vi "Vertical Aiming Calculator.vi"() -> ()   [LabVIEW 2015]
uses:
  <vilib>/Utility/file.llb/Write Delimited Spreadsheet (DBL).vi
panel:
  in  "Robot Constants":T1={"Distance from Pivot Point to Drive Mount(in)"=2.0, "Distance from Pivot Point to Arm Mount(in)"=2.0}
  in  "Other Constants":T2={"Ball Diameter(in)"=10.0, "Air Density(g/in^3)"=0.02, "Drag coefficient"=0.5, "Ball Mass(g)"=300.0, "gravity(in/s^2)"=-386.09, "Minimum Goal Height(in)"=90.0, "Maximum Goal Height(in)"=104.0}
  in  "Sims/angle":i32
  in  "Min Angle":i32
  in  "Max Angle":i32
  in  "Initial Velocity":dbl
  in  "Framerate":i32
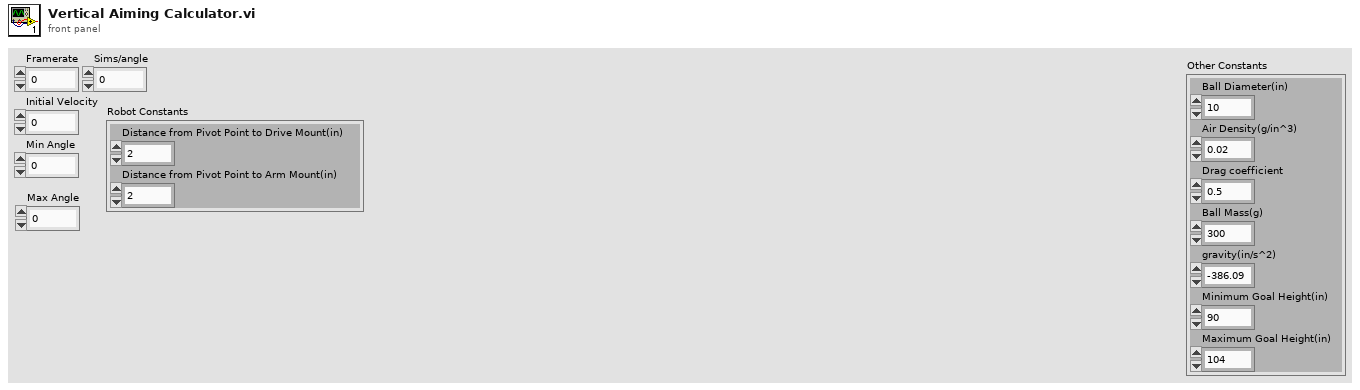
[diagram p1: front panel]
types:
  T1 = cluster{"Distance from Pivot Point to Drive Mount(in)":dbl, "Distance from Pivot Point to Arm Mount(in)":dbl}
  T2 = cluster{"Ball Diameter(in)":dbl, "Air Density(g/in^3)":dbl, "Drag coefficient":dbl, "Ball Mass(g)":dbl, "gravity(in/s^2)":dbl, "Minimum Goal Height(in)":dbl, "Maximum Goal Height(in)":dbl}
  T3 = cluster{"Firing Angle":dbl, "Framerate":dbl, "Initial Velocity":dbl}
  T4 = cluster{"Minimum Distance":dbl, "Ideal Distance":dbl, "Viable Distances":dbl[], "Maximum Distance":dbl}
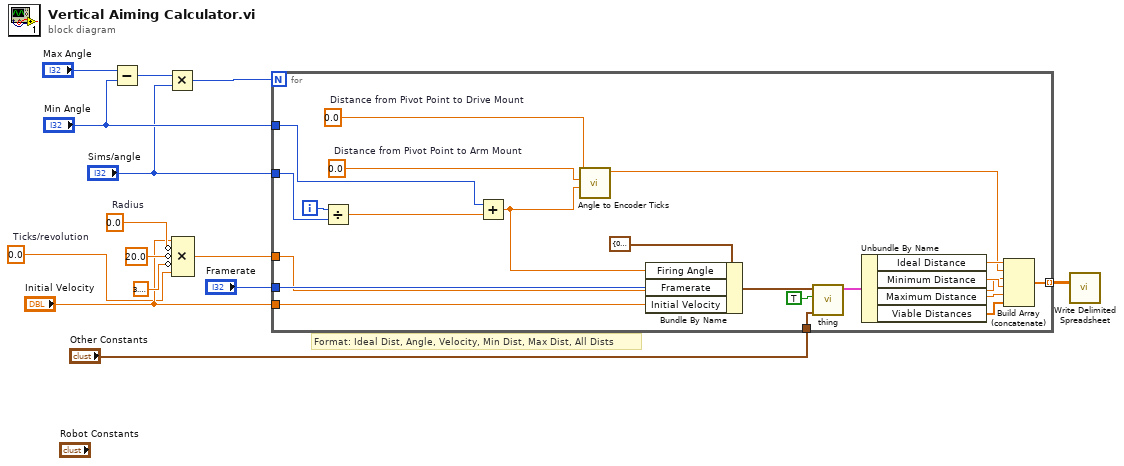
[diagram p0: block diagram]
diagram:
  w3 = 0.0  # Ticks/revolution
  w7 = 0.0  # Radius
  # "Format: Ideal Dist, Angle, Velocity, Min Dist, Max Dist, All Dists"
  n1 = Subtract(x="Max Angle", y="Min Angle") -> (x-y=w10:i32)
  n2 = Multiply(x=w10, y="Sims/angle") -> (x*y=w9:i32)
  n3 = Compound Arithmetic op=MULTIPLY("Initial Velocity", invert w7, invert 20.0 ("value"), invert 3.141592653589793, w3) -> (w2:dbl)
  n4 = for {
    N: w9 -> [_]
    tunnel: "Min Angle" -> [w35]
    tunnel: "Framerate" -> [w32]
    tunnel: "Initial Velocity" -> [w25]
    tunnel: [w29] -> w11 mode=indexing
    tunnel: "Sims/angle" -> [w24]
    tunnel: w2 -> [w17]
    tunnel: "Other Constants" -> [w15]
    i -> [w23]
    w21 = 0.0  # Distance from Pivot Point to Drive Mount
    w19 = 0.0  # Distance from Pivot Point to Arm Mount
    n5 = Divide(x=w23, y=w24) -> (x/y=w22:dbl)
    n6 = Add(x=w35, y=w22) -> (x+y=w20:dbl)
    n7 = call "Angle to Encoder Ticks.vi"("Angle(degrees)"=w20, "Distance from Pivot Point to Arm Mount(in)"=w19, "Distance from Pivot Point to Drive Mount(in)"=w21) -> ("Encoder Ticks"=w18:dbl)  [unwired: 8 in]
    n8 = Bundle By Name(cluster=T3 {"Firing Angle"=0.0, "Framerate"=0.0, "Initial Velocity"=0.0} ("Parameters"), "Firing Angle"=w20, "Framerate"=w32, "Initial Velocity"=w25) -> (w34:T3)
    n9 = call "thing.vi"("Other Constants"=w15, "VisionDistances?"=TRUE, "Parameters"=w34) -> ("Range"=w31:T4)  [unwired: 8 in]
    n10 = Unbundle By Name(w31) -> ("Ideal Distance"=w30:dbl, "Minimum Distance"=w28:dbl, "Maximum Distance"=w27:dbl, "Viable Distances"=w16:dbl[])
    n11 = Build Array (concatenate)(w30, w18, w17, w28, w27, w16) -> (w29:dbl[])
  }
  n12 = call-poly <vilib>:"Write Delimited Spreadsheet.vi"("2D data"=w11) -> ()  [unwired: 13 in, 2 out]
